vi "PPMS.Get Temperature.vi"(8 "error in (no error)":errorcluster, 11 "instrument.PPMS":refnum<class "instrument.PPMS.lvclass">) -> (0 "error out":errorcluster, 2 "Temperature Status":T1, 3 "instrument.PPMS out":refnum<class "instrument.PPMS.lvclass">)   [LabVIEW 2019, in "instrument.PPMS.lvclass"]
uses:
  instrument.PPMS.lvclass
  Typedefs/PPMS.Temperature Status--cluster.ctl
  instrument.PPMS.lvclass/instrument.PPMS.ctl
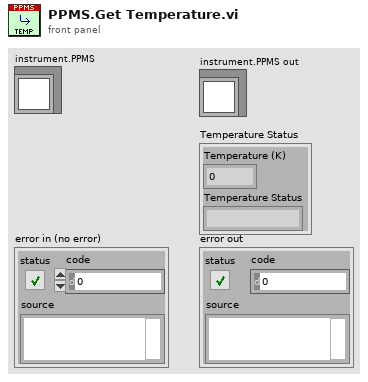
[diagram p1: front panel]
types:
  T1 = typedef "instrument.PPMS.lvclass/PPMS.Temperature Status--cluster.ctl" = cluster{"Temperature (K)":dbl, "Temperature Status":string}
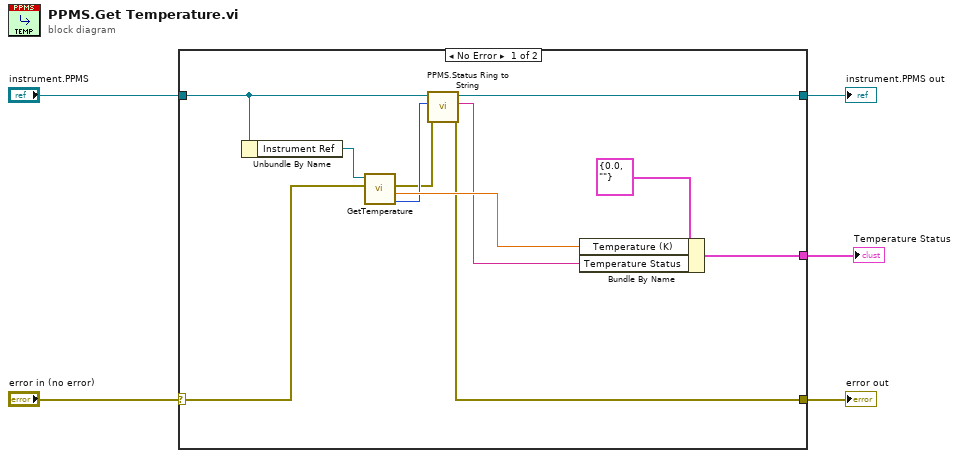
[diagram p0: block diagram]
diagram:
  n1 = case shown="No Error" "error in (no error)" {
    selector: "error in (no error)" -> [w8 w18]
    tunnel: [w7 w18] -> w5
    tunnel: "instrument.PPMS" -> [w10 w17]
    tunnel: [w9 w17] -> w2
    tunnel: [w15 _] -> w1
    frame No Error {
      n2 = Unbundle By Name(w10) -> ("Instrument Ref"=w11:refnum<k24>)
      n3 = call "GetTemperature.vi"("error in (no error)"=w8, "Instrument Ref In"=w11) -> ("Temperature\nStatus"=w14:i32, "Temperature"=w16:dbl, "error out"=w13:errorcluster)  [unwired: 3 in, 2 out]
      n4 = call "PPMS.Status Ring to String.vi"("error in (no error)"=w13, "Temperature Status"=w14, "instrument.PPMS"=w10) -> ("error out"=w7:errorcluster, "Temperature Status String"=w12:string, "instrument.PPMS out"=w9:refnum<class "instrument.PPMS.lvclass">)  [unwired: 5 in, 1 out]
      n5 = Bundle By Name(cluster=T1 {"Temperature (K)"=0.0, "Temperature Status"=""} ("Temperature Status"), "Temperature (K)"=w16, "Temperature Status"=w12) -> (w15:T1)
    }
    frame Error {
    }
  }
  "Temperature Status" <- w1
  "error out" <- w5
  "instrument.PPMS out" <- w2
